vi "Read Displacement Sensors.vi"(8 "error in (no error)":errorcluster, 11 "Model in":refnum<class "Model.lvclass">) -> (0 "error out":errorcluster, 3 "Model out":refnum<class "Model.lvclass">)   [LabVIEW 2016, in "Model.lvclass"]
uses:
  Model.lvclass
  Model.lvclass/Model.ctl
  Common_RT_DLRS1ADisplacementGauge/DLRS1ADisplacementGauge/DLRS1ADisplacementGauge.lvclass/DLRS1ADisplacementGauge.ctl
  common_serialprotocols/SerialProtocol/SerialReal/SerialReal.lvclass
  Common_RT_DLRS1ADisplacementGauge/DLRS1ADisplacementGauge/DLRS1ADisplacementGauge.lvclass
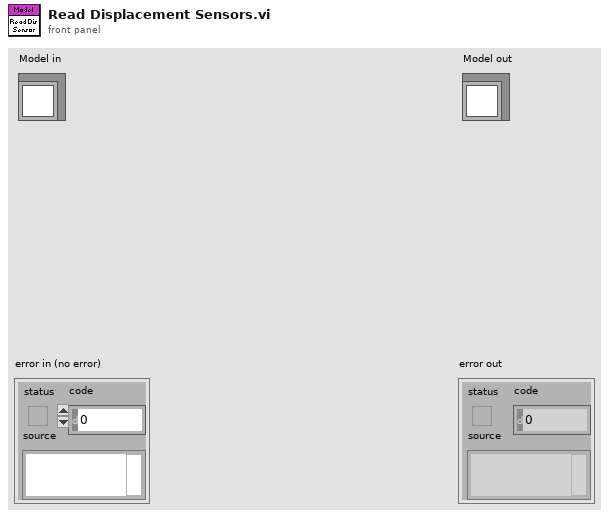
[diagram p1: front panel]
types:
  T1 = typedef "RTDLRS1ADisplacementGauge.lvlib/DLRS1ADisplacementGaugeData.ctl" = cluster{"Telemetry":T2, "Responses":T3}
  T2 = typedef "RTDLRS1ADisplacementGauge.lvlib/DLRS1ADisplacementGaugeTelemetry.ctl" = cluster{"Distance":dbl[]}
  T3 = typedef "RTDLRS1ADisplacementGauge.lvlib/DLRS1ADisplacementGaugeResponses.ctl" = cluster{"Distance":T4}
  T4 = typedef "RTDLRS1ADisplacementGauge.lvlib/DLRS1ADisplacementGaugeErrors.ctl" = enum8{"None", "InvalidCommand", "CommunicationTimeoutError", "DataLengthError", "NumberOfParametersError", "ParameterError", "CommunicationError", "IDNumberError", "ExpansionLineError", "WriteControlError", "UnknownError", "UnknownResponseError"}
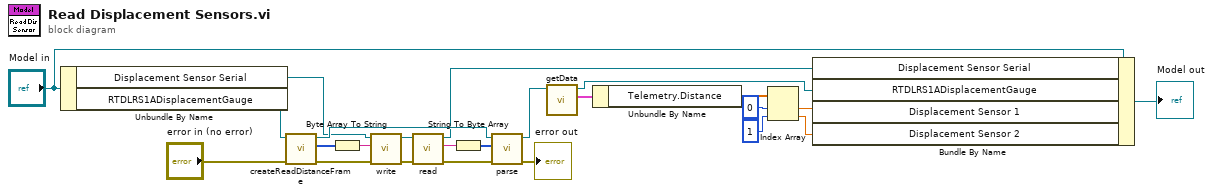
[diagram p0: block diagram]
diagram:
  n1 = Unbundle By Name("Model in") -> ("Displacement Sensor Serial"=w10:refnum<class "SerialReal.lvclass">, "RTDLRS1ADisplacementGauge"=w24:refnum<class "DLRS1ADisplacementGauge.lvclass">)
  n2 = call "createReadDistanceFrame.vi"("error in (no error)"="error in (no error)", "DLRS1ADisplacementGauge in"=w24) -> ("error out"=w14:errorcluster, "Message"=w23:u8[], "DLRS1ADisplacementGauge out"=w11:refnum<class "DLRS1ADisplacementGauge.lvclass">)  [unwired: 7 in]
  n3 = Byte Array To String(unsigned byte array=w23) -> (string=w22:string)
  n4 = call-dynamic "write.vi"("error in (no error)"=w14, "writeString"=w22, "SerialReal in"=w10) -> ("error out"=w20:errorcluster, "SerialReal out"=w21:refnum<class "SerialReal.lvclass">)  [unwired: 7 in]
  n5 = call-dynamic "read.vi"("error in (no error)"=w20, "SerialReal in"=w21) -> ("error out"=w13:errorcluster, "stringRead"=w19:string, "SerialReal out"=w9:refnum<class "SerialReal.lvclass">)  [unwired: 7 in]
  n6 = String To Byte Array(string=w19) -> (unsigned byte array=w18:u8[])
  n7 = call "parse.vi"("error in (no error)"=w13, "Message"=w18, "DLRS1ADisplacementGauge in"=w11) -> ("error out"=→"error out":errorcluster, "DLRS1ADisplacementGauge out"=w8:refnum<class "DLRS1ADisplacementGauge.lvclass">)  [unwired: 6 in, 1 out]
  n8 = call "getData.vi"("DLRS1ADisplacementGauge in"=w8) -> ("DLRS1ADisplacementGaugeData"=w7:T1, "DLRS1ADisplacementGauge out"=w1:refnum<class "DLRS1ADisplacementGauge.lvclass">)  [unwired: 9 in]
  n9 = Unbundle By Name(w7) -> ("Telemetry.Distance"=w6:dbl[])
  n10 = Index Array(array=w6, index #1=0 ("index"), index #2=1 ("index")) -> (element #1=w3:dbl, element #2=w2:dbl)
  n11 = Bundle By Name(cluster="Model in", "Displacement Sensor Serial"=w9, "RTDLRS1ADisplacementGauge"=w1, "Displacement Sensor 1"=w3, "Displacement Sensor 2"=w2) -> (→"Model out":refnum<class "Model.lvclass">)
